vi "FlexRay_Value_Analysis.vi"(10 "FDatas":u8[](array[numeric]), 11 "TFlexRaySignal":T1) -> (3 "Signal Value":dbl)   [LabVIEW 2014]
uses:
  Typedef/FlexRay/TFlexRaySignal.ctl
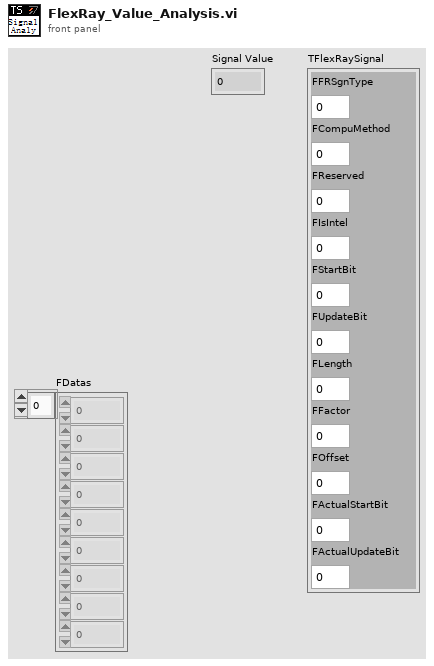
[diagram p1: front panel]
types:
  T1 = typedef "TFlexRaySignal.ctl" = cluster{"FFRSgnType":u8, "FCompuMethod":u8, "FReserved":u8, "FIsIntel":u8, "FStartBit":i32, "FUpdateBit":i32, "FLength":i32, "FFactor":dbl, "FOffset":dbl, "FActualStartBit":i32, "FActualUpdateBit":i32}
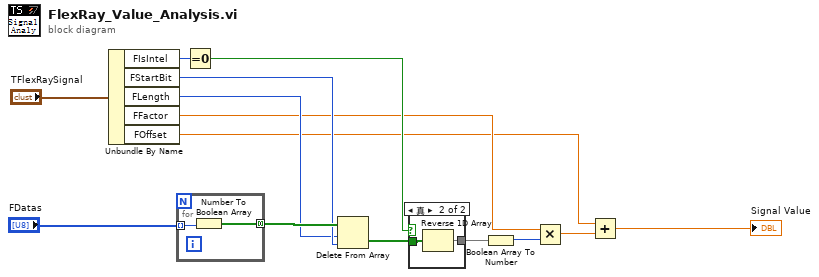
[diagram p0: block diagram]
diagram:
  n1 = Unbundle By Name("TFlexRaySignal") -> ("FIsIntel"=w5:u8, "FStartBit"=w4:i32, "FLength"=w3:i32, "FFactor"=w2:dbl, "FOffset"=w1:dbl)
  n2 = for {
    tunnel: "FDatas" -> [w16] mode=indexing
    tunnel: [w15] -> w9 mode=concatenating
    n3 = Number To Boolean Array(number=w16) -> (Boolean array=w15:bool[])
  }
  n4 = Equal To 0?(x=w5) -> (x = 0?=w10:bool)
  n5 = Delete From Array(array=w9, length=w3, index=w4) -> (deleted portion=w7:bool[])  [unwired: 1 out]
  n6 = case shown="真" w10 {
    tunnel: w7 -> [w17 w19]
    tunnel: [w17 w18] -> w11
    frame False {
    }
    frame True {
      n7 = Reverse 1D Array(array=w19) -> (reversed array=w18:bool[])
    }
  }
  n8 = Boolean Array To Number(Boolean array=w11) -> (number=w12:u32)
  n9 = Multiply(x=w2, y=w12) -> (x*y=w13:dbl)
  n10 = Add(x=w1, y=w13) -> (x+y=→"Signal Value":dbl)
